vi "Template.vi"() -> ()   [LabVIEW 2014]
uses:
  02_Controls/Message_Queues.ctl
  02_Controls/Message_Data_Ctl.ctl
panel:
  in  "Message_Queues":T1
  out "error out":errorcluster
  in  "error in (no error)":errorcluster
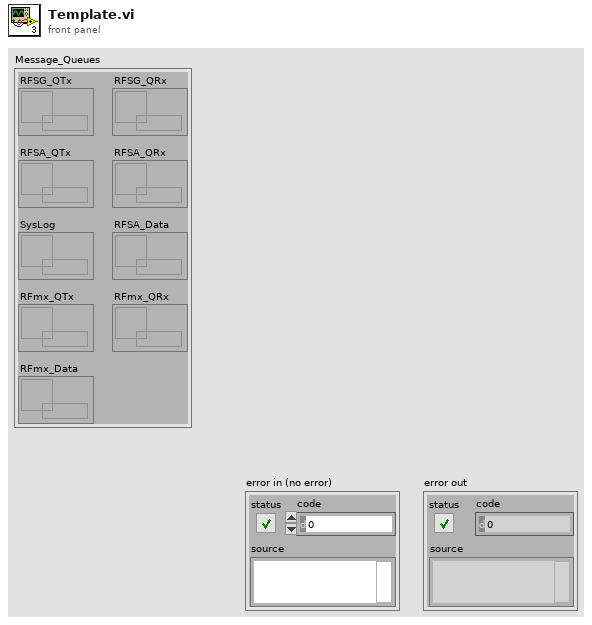
[diagram p1: front panel]
types:
  T1 = typedef "Message_Queues.ctl" = cluster{"RFSG_QTx":refnum<queue>, "RFSG_QRx":refnum<queue>, "RFSA_QTx":refnum<queue>, "RFSA_QRx":refnum<queue>, "SysLog":refnum<queue>, "RFSA_Data":refnum<queue>, "RFmx_QTx":refnum<queue>, "RFmx_QRx":refnum<queue>, "RFmx_Data":refnum<queue>}
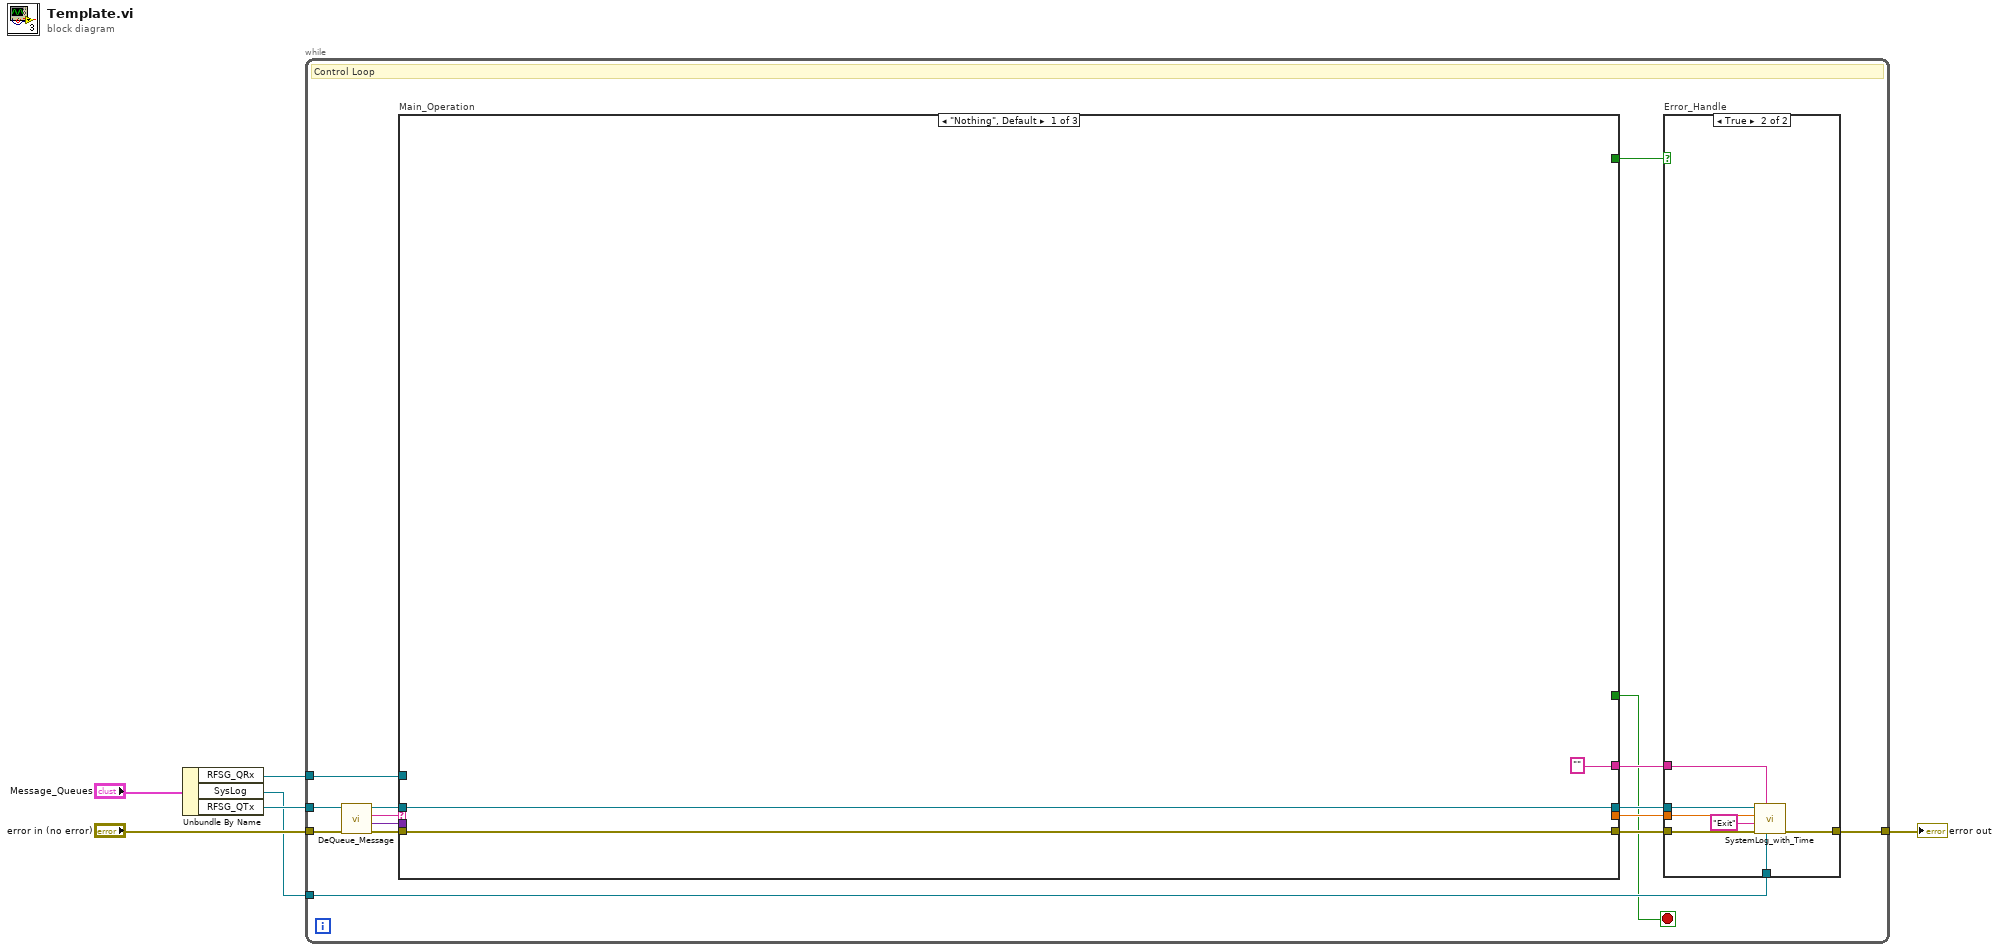
[diagram p0: block diagram]
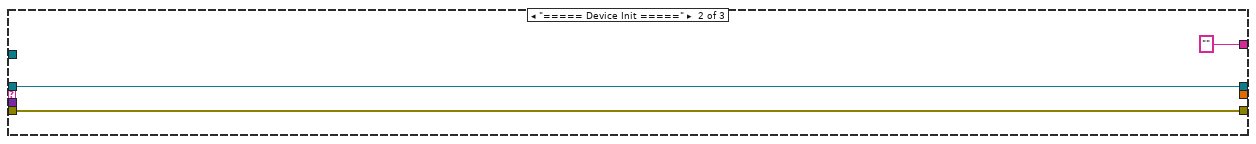
[diagram p3: hidden frame]
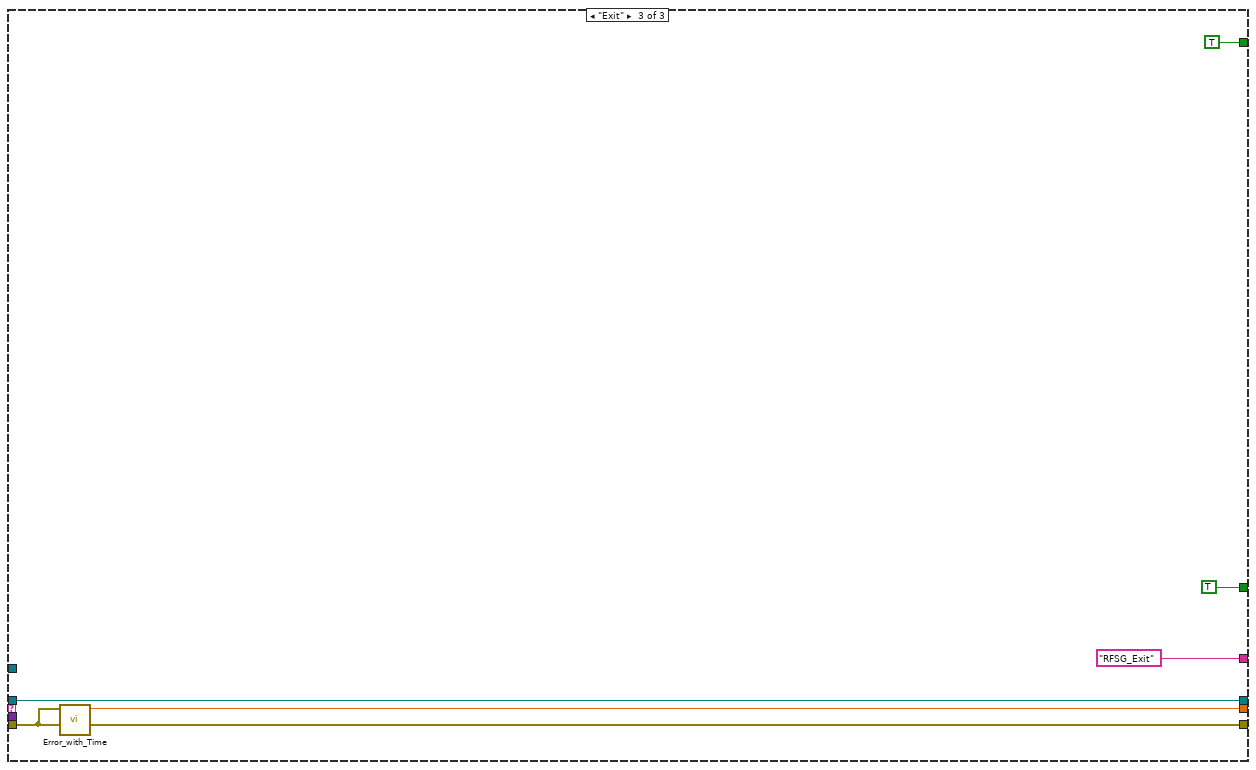
[diagram p4: hidden frame]
diagram:
  n1 = Unbundle By Name("Message_Queues") -> ("RFSG_QRx"=w2:refnum<queue>, "SysLog"=w1:refnum<queue>, "RFSG_QTx"=w4:refnum<queue>)
  n2 = while {
    tunnel: "error in (no error)" -> [w21]
    tunnel: [w14] -> w5
    tunnel: w4 -> [w16]
    tunnel: w2 -> [w15]
    tunnel: w1 -> [w9]
    stop <- w8 stop-if-true
    # "Control Loop"
    n3 = call "DeQueue_Message.vi"("error in (no error)"=w21, "Message_Queue"=w16) -> ("error out"=w17:errorcluster, "Message Data"=w19:variant, "Message"=w20:string, "Dup_Message_Queue"=w18:refnum<queue>)  [unwired: 6 in]
    n4 = case "Main_Operation" shown="\"Nothing\", Default" w20 {
      tunnel: w19 -> [_ _ _]
      tunnel: w18 -> [w30 w33 w39]
      tunnel: w17 -> [w32 w35 w36]
      tunnel: [_ _ TRUE] -> w8
      tunnel: [w32 w35 w36] -> w12
      tunnel: w15 -> [_ _ _]
      tunnel: ["" ("Message") "" ("Message") "RFSG_Exit" ("Message")] -> w13
      tunnel: [_ _ w37] -> w11
      tunnel: [w30 w33 w39] -> w10
      tunnel: [_ _ TRUE] -> w7
      frame "Nothing", Default {
      }
      frame "===== Device Init =====" {
      }
      frame "Exit" {
        n5 = call "Error_with_Time.vi"("error in (no error)"=w36) -> ("relative seconds"=w37:dbl)  [unwired: 10 in]
      }
    }
    n6 = case "Error_Handle" shown="True" w7 {
      tunnel: w12 -> [w22 w29]
      tunnel: [w22 w28] -> w14
      tunnel: w13 -> [_ w27]
      tunnel: w10 -> [_ w26]
      tunnel: w11 -> [_ w25]
      tunnel: w9 -> [_ w24]
      frame False {
      }
      frame True {
        n7 = call "SystemLog_with_Time.vi"("SysLog_Queue"=w24, "Message_in"=w27, "error in (no error)"=w29, "Send_Msg"="Exit", "Tick_in"=w25, "Worker_Queue"=w26) -> ("error out"=w28:errorcluster)  [unwired: 5 in]
      }
    }
  }
  "error out" <- w5
